vi "Firmware Wizard Check INI.vi"(8 "Error In":errorcluster) -> (0 "Error Out":errorcluster)   [LabVIEW 2013, in "LVH-LINX.lvlib"]
uses:
  <vilib>/LabVIEW Hacker/LINX/LVH-LINX.lvlib
  <vilib>/Utility/config.llb/NI_LVConfig.lvlib
  <vilib>/Utility/config.llb/Write Key (Path).vi
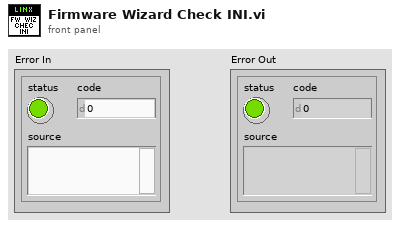
[diagram p1: front panel]
types:
  T1 = typedef "NI_LVConfig.lvlib/Config Data RefNum.ctl" = refnum<k1>
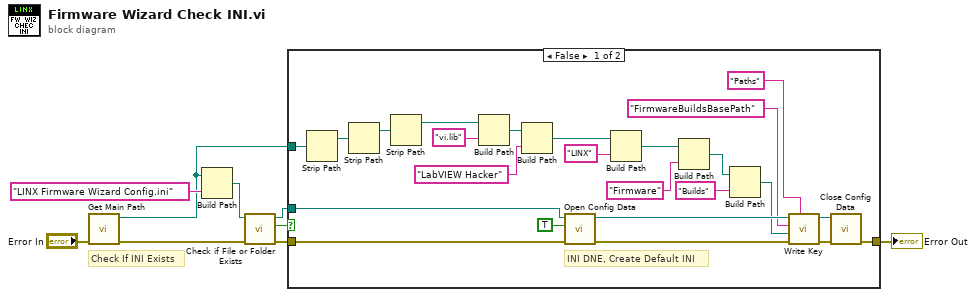
[diagram p0: block diagram]
diagram:
  # "Check If INI Exists"
  n1 = call <vilib>:"Get Main Path.vi"("Error In"="Error In") -> ("Error Out"=w9:errorcluster, "Main Dir"=w2:path)  [unwired: 8 in, 1 out]
  n2 = Build Path(base path=w2, name or relative path="LINX Firmware Wizard Config.ini") -> (appended path=w6:path)
  n3 = call <vilib>:"Check if File or Folder Exists.vi"("error in (no error)"=w9, "path"=w6) -> ("error out"=w5:errorcluster, "file or folder exists?"=w4:bool, "dup path"=w1:path)  [unwired: 7 in]
  n4 = case shown="False" w4 {
    tunnel: w5 -> [w26 w34]
    tunnel: [w20 w34] -> w3
    tunnel: w2 -> [w25 _]
    tunnel: w1 -> [w19 _]
    frame False {
      # "INI DNE, Create Default INI"
      n5 = Strip Path(path=w25) -> (stripped path=w18:path)  [unwired: 1 out]
      n6 = Strip Path(path=w18) -> (stripped path=w17:path)  [unwired: 1 out]
      n7 = Strip Path(path=w17) -> (stripped path=w16:path)  [unwired: 1 out]
      n8 = Build Path(base path=w16, name or relative path="vi.lib") -> (appended path=w14:path)
      n9 = Build Path(base path=w14, name or relative path="LabVIEW Hacker") -> (appended path=w12:path)
      n10 = call <vilib>:"Open Config Data.vi"("error in (no error)"=w26, "create file if necessary (T)"=TRUE, "configuration file path"=w19) -> ("error out"=w31:errorcluster, "refnum"=w30:T1)  [unwired: 6 in, 1 out]
      n11 = Build Path(base path=w12, name or relative path="LINX") -> (appended path=w10:path)
      n12 = Build Path(base path=w10, name or relative path="Firmware") -> (appended path=w22:path)
      n13 = Build Path(base path=w22, name or relative path="Builds") -> (appended path=w21:path)
      n14 = call-poly <vilib>:"Write Key.vi"("section"="Paths", "error in (no error)"=w31, "value"=w21, "key"="FirmwareBuildsBasePath", "refnum"=w30) -> ("error out"=w32:errorcluster, "refnum out"=w33:T1)  [unwired: 4 in, 1 out]
      n15 = call <vilib>:"Close Config Data.vi"("error in (no error)"=w32, "refnum"=w33) -> ("error out"=w20:errorcluster)  [unwired: 8 in, 1 out]
    }
    frame True {
      # "INI Exists, Nothing To Do"
    }
  }
  "Error Out" <- w3
